vi "Write-Read_txt.vi"() -> ()   [LabVIEW 2010]
doc: "This example shows how the Write and Read Text File functions operate using different options. Click the Run button to execute and examine the behavior of each case."
panel:
  in  "stop":bool
  in  "Tab Control":T1(tab)
  in  "Choose":string(combo)
  in  "Path":path=path "C:/write-read example.txt"
  in  "Write Text 2":string="This text will be\nwritten to file."
  out "Read Text 2":string
  in  "Path":path
  out "Read Text":string
  in  "Write Text":string="This text will be\nwritten to file."
  in  "Path":path
  in  "Write Text":string="This text will be\\n\nwritten to file.\\n\\r"
  out "Read Text":string
  in  "Path":path
  out "Read Text":string
  in  "Write Text":string="This text will be\nwritten to file."
  in  "Path":path
  in  "Count":i32=-1
  out "Read Text Array":string[](array[string])
  in  "Write Text":string="This text will be\nwritten to file."
  # "This example shows how the Write and Read Text File \nfunctions operate using different options.  Click the Run \nbutton to execute and examine the behavior of each case."
  # "Both the Write and Read Text File functions \ncan identify files using a path.  This case shows \nhow the functions will execute when a path is defined."
  # "The Write and Read Text File functions can also \nidentify files using the file refnum, provided by \nthe Open/Create/Replace function."
  # "By default, LabVIEW Converts the EOL characters \ndepending on the platform.  In this case the EOL \nConvert option has been disabled on the Write and \nRead Text File by right-clicking on the function and \nunchecking that option.  Notice that the text file \nthat is created does not have the proper formatting."
  # "The Read Lines option will allow the Read Text File function \nto read lines instead of characters.  In this case the Read \nLines function has been enabled by right-clicking the Read \nText File function and checking that option.  Notice that \nonly one line is read by default."
  # "This case also enables the Read Lines option, but uses \nthe Count input to the Read Text File function, which \ndefines the number of lines to read.  This causes the \noutput of the function to be an array of strings, each \nelement corresponding to a line.  The Count parameter \ncan be set to -1 to read the entire file."
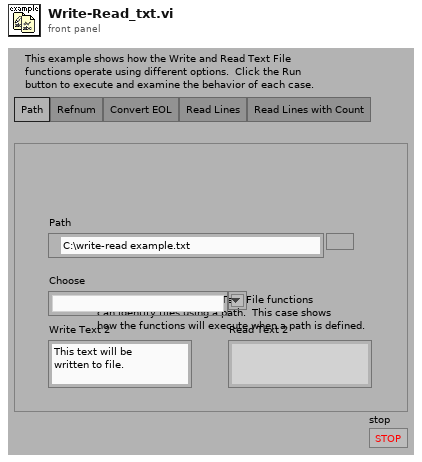
[diagram p1: front panel]
types:
  T1 = enum32{"Path", "Refnum", "Convert EOL", "Read Lines", "Read Lines with Count"}
  T2 = enum16{"open", "replace", "create", "open or create", "replace or create", "replace or create with confirmation"}
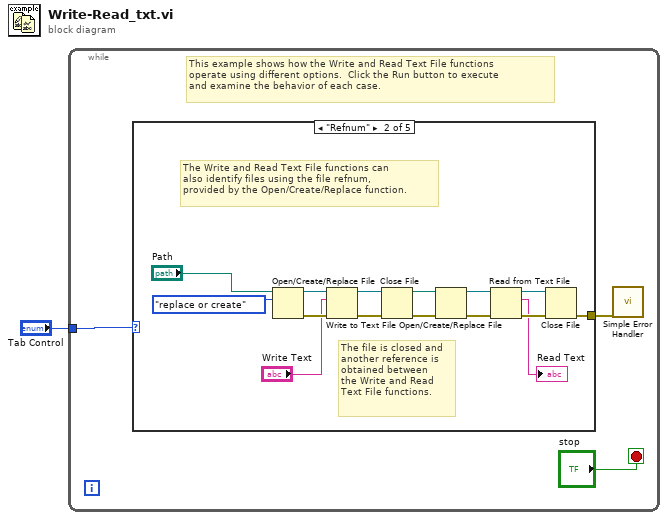
[diagram p0: block diagram]
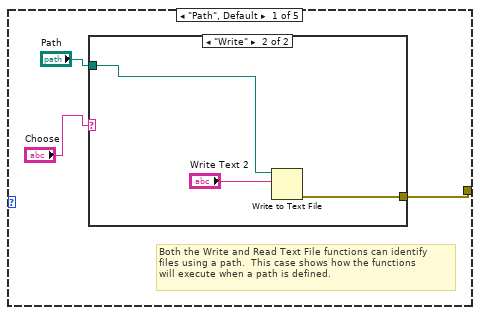
[diagram p2: hidden frame]
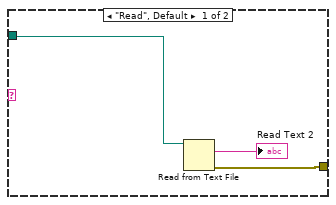
[diagram p3: hidden frame]
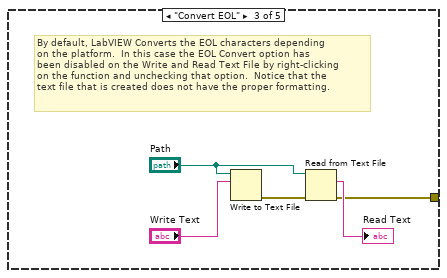
[diagram p4: hidden frame]
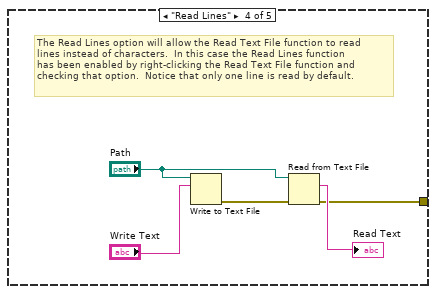
[diagram p5: hidden frame]
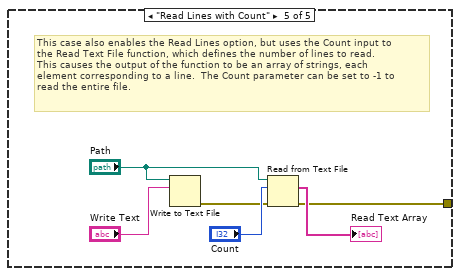
[diagram p6: hidden frame]
diagram:
  n1 = while {
    tunnel: "Tab Control" -> [w4]
    stop <- "stop" stop-if-true
    # "This example shows how the Write and Read Text File functions \noperate using different options.  Click the Run button to execute \nand examine the behavior of each case."
    n2 = case shown="\"Refnum\"" w4 {
      tunnel: [w6 w23 w30 w35 w40] -> w3
      frame "Path", Default {
        # "Both the Write and Read Text File functions can identify \nfiles using a path.  This case shows how the functions \nwill execute when a path is defined."
        n3 = case shown="\"Write\"" "Choose" {
          tunnel: "Path" -> [w9 w13]
          tunnel: [w8 w12] -> w6
          frame "Read", Default {
            n4 = Read from Text File(file (use dialog)=w9) -> (text=→"Read Text 2":string, error out=w8:errorcluster)  [unwired: 3 in, 2 out]
          }
          frame "Write" {
            n5 = Write to Text File(file (use dialog)=w13, text="Write Text 2") -> (error out=w12:errorcluster)  [unwired: 2 in, 2 out]
          }
        }
      }
      frame "Refnum" {
        # "The Write and Read Text File functions can \nalso identify files using the file refnum, \nprovided by the Open/Create/Replace function."
        # "The file is closed and \nanother reference is \nobtained between \nthe Write and Read \nText File functions."
        n6 = Open/Create/Replace File(file path (use dialog)="Path", operation (0:open)=T2."replace or create") -> (refnum out=w26:refnum<file>, error out=w28:errorcluster)  [unwired: 4 in, 1 out]
        n7 = Write to Text File(file (use dialog)=w26, text="Write Text", error in=w28) -> (refnum out=w20:refnum<file>, error out=w16:errorcluster)  [unwired: 1 in, 1 out]
        n8 = Close File(refnum=w20, error in=w16) -> (path=w19:path, error out=w18:errorcluster)
        n9 = Open/Create/Replace File(file path (use dialog)=w19, error in=w18) -> (refnum out=w17:refnum<file>, error out=w15:errorcluster)  [unwired: 4 in, 1 out]
        n10 = Read from Text File(file (use dialog)=w17, error in=w15) -> (refnum out=w25:refnum<file>, text=→"Read Text":string, error out=w24:errorcluster)  [unwired: 2 in, 1 out]
        n11 = Close File(refnum=w25, error in=w24) -> (error out=w23:errorcluster)  [unwired: 1 out]
      }
      frame "Convert EOL" {
        # "By default, LabVIEW Converts the EOL characters depending \non the platform.  In this case the EOL Convert option has \nbeen disabled on the Write and Read Text File by right-clicking \non the function and unchecking that option.  Notice that the \ntext file that is created does not have the proper formatting."
        n12 = Write to Text File(file (use dialog)="Path", text="Write Text") -> (error out=w31:errorcluster)  [unwired: 2 in, 2 out]
        n13 = Read from Text File(file (use dialog)="Path", error in=w31) -> (text=→"Read Text":string, error out=w30:errorcluster)  [unwired: 2 in, 2 out]
      }
      frame "Read Lines" {
        # "The Read Lines option will allow the Read Text File function to read \nlines instead of characters.  In this case the Read Lines function \nhas been enabled by right-clicking the Read Text File function and \nchecking that option.  Notice that only one line is read by default."
        n14 = Write to Text File(file (use dialog)="Path", text="Write Text") -> (error out=w36:errorcluster)  [unwired: 2 in, 2 out]
        n15 = Read from Text File(file (use dialog)="Path", error in=w36) -> (text=→"Read Text":string, error out=w35:errorcluster)  [unwired: 2 in, 2 out]
      }
      frame "Read Lines with Count" {
        # "This case also enables the Read Lines option, but uses the Count input to \nthe Read Text File function, which defines the number of lines to read.  \nThis causes the output of the function to be an array of strings, each \nelement corresponding to a line.  The Count parameter can be set to -1 to \nread the entire file."
        n16 = Write to Text File(file (use dialog)="Path", text="Write Text") -> (error out=w41:errorcluster)  [unwired: 2 in, 2 out]
        n17 = Read from Text File(file (use dialog)="Path", count="Count", error in=w41) -> (text=→"Read Text Array":string[], error out=w40:errorcluster)  [unwired: 1 in, 2 out]
      }
    }
    n18 = call <vilib>:"Simple Error Handler.vi"("error in (no error)"=w3) -> ()  [unwired: 4 in, 5 out]
  }
